vi "AMI_ScanCampo Y axis.vi"(6 "error in (no error)":errorcluster, 7 "Index":i8) -> (0 "error out":errorcluster, 1 "resulting string 2":string="End scan field", 2 "resulting string 1":string="Scan Field from 0.000Tesla to 0.500Tesla at 1.000Tesla/min, in 50 steps, Driven")   [LabVIEW 2017]
doc: "Use this template to create a dialog box. This template polls the state of the buttons on the front panel and does not use events. Use the Dialog Using Events template (not available in Base package) to create a dialog box with event handling."
panel:
  in  "# puntos":u16
  in  "Campo Final (T)":dbl=0.1 min=-2.0 max=2.0 format="%.3f"
  in  "Modo de barrido":i32(ring) items=["Solo ir", "Ir y volver"]
  out "Y Ramp Units":u16(ring)=1 items=["Per SECOND", "Per MINUTE"]
  out "Y Field Units":u16(ring)=1 items=["KGauss", "Tesla"]
  out "Wait stability":bool=TRUE
  in  "Rate (T/min)":dbl=0.03 min=0.0 max=0.1 step=0.001 format="%.3f"
  in  "Campo Inicial (T)":dbl min=-2.0 max=2.0 format="%.3f"
  out "Cancelled?":bool
  in  "Cancel":bool
  in  "OK":bool
  # "SCAN Y MAGNETIC FIELD"
  # "Nov 2022 V2.1  a-sslcdms"
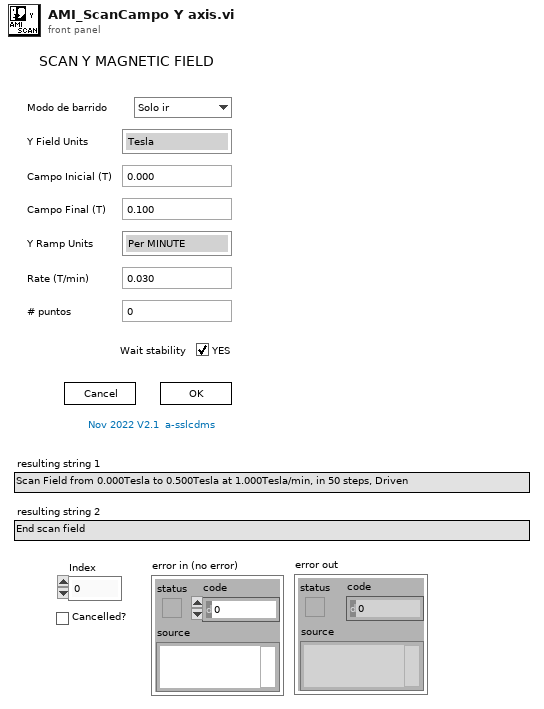
[diagram p1: front panel]
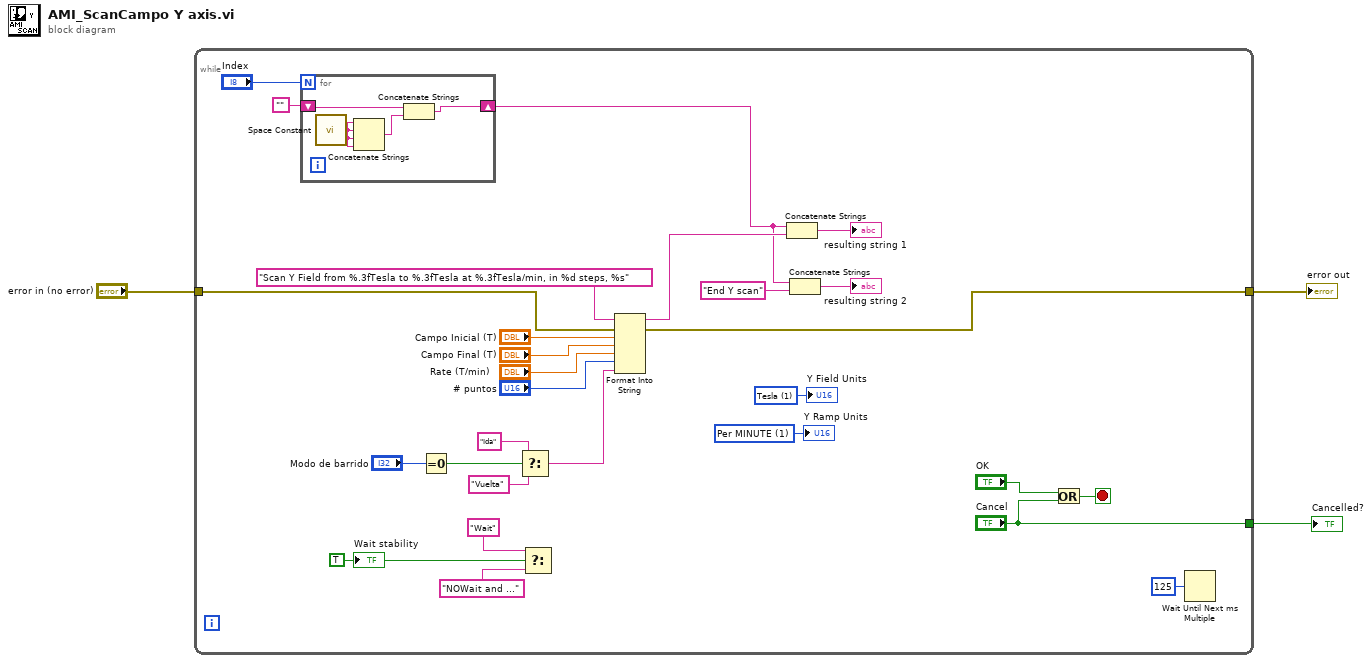
[diagram p0: block diagram]
diagram:
  n1 = while {
    tunnel: ["Cancel"] -> w3
    tunnel: [w5] -> w2
    tunnel: "error in (no error)" -> [w6]
    stop <- w30 stop-if-true
    w21 = u16 1 items=["Per SECOND", "Per MINUTE"] ("Ramp Units")
    w22 = u16 1 items=["KGauss", "Tesla"] ("Field Units")
    w25 = TRUE ("Wait stability")
    n2 = for {
      N: "Index" -> [_]
      shift-right: [w34] -> w4
      shift-left: "" -> [w33]
      n3 = call <vilib>:"Space Constant.vi"() -> ("String"=w32:string)
      n4 = Concatenate Strings(w32, w32, w32, w32) -> (w35:string)
      n5 = Concatenate Strings(w33, w35) -> (w34:string)
    }
    n6 = Equal To 0?(x="Modo de barrido") -> (x = 0?=w17:bool)
    n7 = Select(t="Ida" ("resulting string 2"), s=w17, f="Vuelta" ("resulting string 2")) -> (s? t:f=w16:string)
    n8 = Select(t="Wait", s=w25, f="NOWait and ...") -> ()  [unwired: 1 out]
    n9 = Format Into String(format string="Scan Y Field from %.3fTesla to %.3fTesla at %.3fTesla/min, in %d steps, %s", error in=w6, "Campo Inicial (T)", "Campo Final (T)", "Rate (T/min)", "# puntos", w16) -> (resulting string=w20:string, error out=w5:errorcluster)  [unwired: 1 in]
    n10 = Concatenate Strings(w4, w20) -> (→"resulting string 1":string)
    n11 = Concatenate Strings(w4, "End Y scan" ("resulting string 2")) -> (→"resulting string 2":string)
    n12 = Or(x="OK", y="Cancel") -> (x .or. y?=w30:bool)
    n13 = Wait Until Next ms Multiple(millisecond multiple=u32 125) -> ()  [unwired: 1 out]
    "Wait stability" <- w25
    "Y Field Units" <- w22
    "Y Ramp Units" <- w21
  }
  "Cancelled?" <- w3
  "error out" <- w2
